vi "listeTachesProjet.vi"(1 "Id Personnel":string, 2 "Id Projet":string) -> (0 "Liste Tâches":string[][](table))   [LabVIEW 2024]
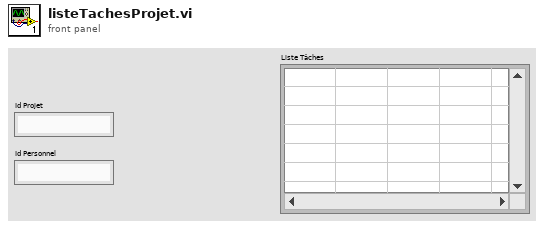
[diagram p1: front panel]
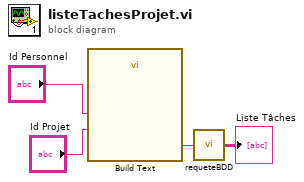
[diagram p0: block diagram]
diagram:
  n1 = call "Build Text"("id_personnel"="Id Personnel", "id_projet"="Id Projet") -> ("Result"=w2:string)  [unwired: 12 in, 1 out]
  n2 = call "requeteBDD.vi"("Requête Sql"=w2) -> ("Table Control"=→"Liste Tâches":string[][])
